vi "execute.vi"(8 "error in (no error)":errorcluster, 10 "ComponentData.lvclass":refnum<class "ComponentData.lvclass">, 11 "FaultState in":refnum<class "FaultState.lvclass">) -> (0 "error out":errorcluster, 2 "ComponentData.lvclass 2":refnum<class "ComponentData.lvclass">, 3 "FaultState out":refnum<class "FaultState.lvclass">)   [LabVIEW 2013, in "ComponentData.lvlib" / "FaultState.lvclass"]
uses:
  <userlib>/Common/Component/Application/RT/ComponentData/ComponentState/FaultState/FaultState.lvclass
  <userlib>/Common/Component/Application/RT/ComponentData/ComponentData/ComponentData.lvclass
  <userlib>/Common/Component/Application/RT/ComponentData/ComponentState/ComponentState/ComponentState.lvclass
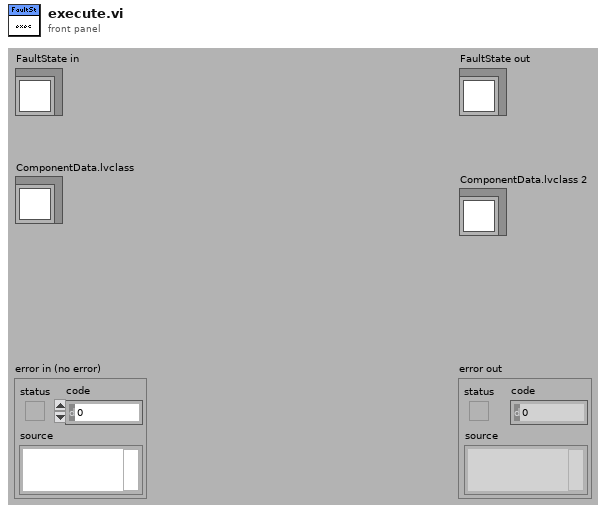
[diagram p1: front panel]
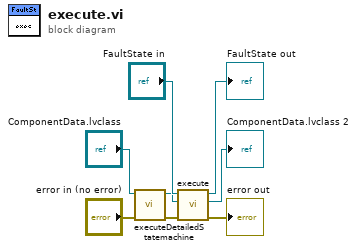
[diagram p0: block diagram]
diagram:
  n1 = call-dynamic "executeDetailedStatemachine.vi"("error in (no error)"="error in (no error)", "ComponentData in"="ComponentData.lvclass") -> ("error out"=w1:errorcluster, "ComponentData out"=w3:refnum<class "ComponentData.lvclass">)  [unwired: 8 in]
  n2 = call-parent "execute.vi"("error in (no error)"=w1, "ComponentData.lvclass"=w3, "ComponentState in"="FaultState in") -> ("error out"=→"error out":errorcluster, "ComponentData.lvclass 2"=→"ComponentData.lvclass 2":refnum<class "ComponentData.lvclass">, "ComponentState out"=→"FaultState out":refnum<class "FaultState.lvclass">)  [unwired: 6 in]
